vi "MT Apply Matched Filter (MSK).vi"(0 "input complex waveform":T1={"t0"=0.0, "dt"=1.0, "Y"=[]} {"Y" format="%.3f"; "dt" format="%^.2e"; "t0" format="%.4f"}, 5 "matched filter coefficients":dbl[](array[numeric]) format="%^.2e", 7 "samples per symbol (16)":i32=16, 11 "error in (no error)":errorcluster, 13 "reset? (T)":bool=TRUE) -> (4 "output phase waveform":cluster{"t0":dbl, "dt":dbl, "Y":dbl[]} {"Y" min=0.0 max=127.0 format="%.3f"; "dt" format="%^.2e"; "t0" format="%.4f"}, 15 "error out":errorcluster)   [LabVIEW 2020, in "niDMT.lvlib"]
doc: "This polymorphic instance applies a matched filter to an input MSK-modulated waveform. The VI first performs phase differentiation, followed by matched filtering on the phase of the <B>input complex waveform</B>."
uses:
  <vilib>/addons/Modulation/niDMT.lvlib
  <vilib>/addons/Modulation/Analog/controls/Complex Data Waveform.ctl
  <vilib>/addons/Modulation/niAMT.lvlib
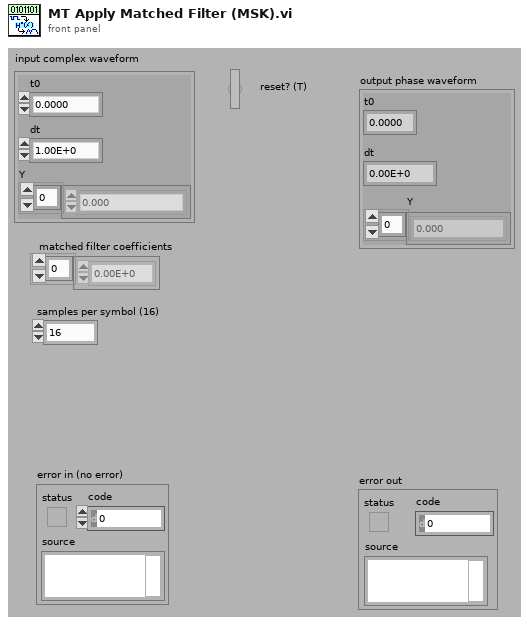
[diagram p1: front panel]
types:
  T1 = typedef "niAMT.lvlib/Complex Data Waveform.ctl" = cluster{"t0":dbl, "dt":dbl, "Y":cdb[]}
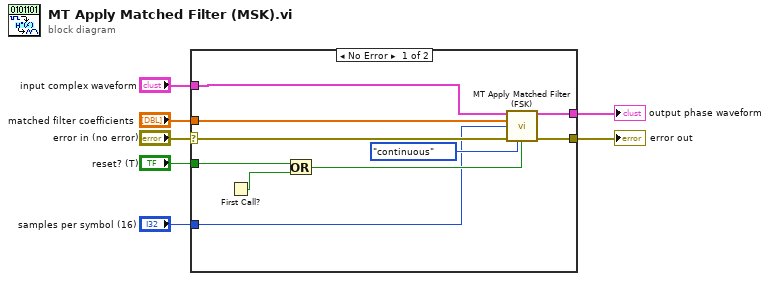
[diagram p0: block diagram]
diagram:
  n1 = case shown="No Error" "error in (no error)" {
    selector: "error in (no error)" -> [w10 w18]
    tunnel: "input complex waveform" -> [w9 _]
    tunnel: [w17 w18] -> w2
    tunnel: "matched filter coefficients" -> [w16 _]
    tunnel: "reset? (T)" -> [w15 _]
    tunnel: [w12 _] -> w3
    tunnel: "samples per symbol (16)" -> [w8 _]
    frame No Error {
      n2 = First Call?() -> (First Call?: T/F=w14:bool)
      n3 = Or(x=w15, y=w14) -> (x .or. y?=w13:bool)
      n4 = call <vilib>:"MT Apply Matched Filter (FSK).vi"("input complex waveform"=w9, "matched filter coefficients"=w16, "samples per symbol (16)"=w8, "error in (no error)"=w10, "symbol phase continuity"=enum16{"continuous", "discontinuous"}."continuous", "reset? (T)"=w13) -> ("output phase waveform"=w12:cluster{"t0":dbl, "dt":dbl, "Y":dbl[]}, "error out"=w17:errorcluster)  [unwired: 1 in, 7 out]
    }
    frame Error {
    }
  }
  "output phase waveform" <- w3
  "error out" <- w2
